vi "ShoulderBegin.vi"(8 "error in (no error)":errorcluster) -> (0 "error out":errorcluster)   [LabVIEW 2023]
doc: "Arm begin\nOpens ArmLift motor\nInputs:\nNone\nOutputs:\nnone"
uses:
  <vilib>/Rock Robotics/WPI/ThirdParty/REV Robotics/REVLib/Typedef/Spark MAX Sensor Type.ctl
  <vilib>/Rock Robotics/WPI/ThirdParty/REV Robotics/REVLib/Typedef/Spark MAX Limit Direction.ctl
  <vilib>/Rock Robotics/WPI/ThirdParty/REV Robotics/REVLib/Typedef/Spark MAX Limit Switch Polarity.ctl
  <vilib>/Rock Robotics/WPI/ThirdParty/REV Robotics/REVLib/Typedef/Spark MAX Idle Mode.ctl
  <vilib>/Rock Robotics/WPI/ThirdParty/REV Robotics/REVLib/Typedef/Spark MAX Motor Type.ctl
  <vilib>/Rock Robotics/WPI/Switch/WPI_SwitchOpenLimit.vi
  <vilib>/Rock Robotics/SystemInterfaces/DIO/FPGA_DIOChannel.ctl
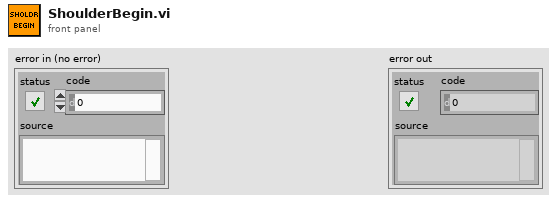
[diagram p1: front panel]
types:
  T1 = typedef "Spark MAX Sensor Type.ctl" = enum16{"No Sensor", "Hall Sensor", "Encoder", "-Not Available-", "Analog", "Alternate Encoder", "Duty Cycle"}
  T2 = typedef "Spark MAX Limit Switch Polarity.ctl" = enum16{"Normally Open", "Normally Closed"}
  T3 = typedef "Spark MAX Limit Direction.ctl" = enum16{"Forward Limit", "Reverse Limit"}
  T4 = typedef "Spark MAX Idle Mode.ctl" = enum16{"Coast", "Brake"}
  T5 = typedef "Spark MAX Motor Type.ctl" = enum16{"Brushed", "Brushless"}
  T6 = typedef "WPI_MotorControlDeviceRef.ctl" = cluster{"DeviceStatus":errorcluster, "Type":T7, "PWM":cluster{"PWM Channel":T8, "DeadBand":T9}, "CAN":cluster{"Device Number":u8, "SetOutput VI Ref":variant, "GetOutput VI Ref":variant, "Enable VI Ref":variant, "Disable VI Ref":variant, "Data":variant}, "Invert":bool, "DIO PWM":cluster{"PWM \"Enable\" Channel":T8, "DIOChannel":T10, "PWM Rate":dbl}}
  T7 = typedef "WPI_MotorControlType.ctl" = enum16{"PWM", "CAN", "DIO PWM"}
  T8 = typedef "FPGA_DIOPWMChannel.ctl" = enum8{"PWM 0", "PWM 1", "PWM 2", "PWM 3", "PWM 4", "PWM 5", "PWM 6", "PWM 7", "PWM 8", "PWM 9", "PWM MXP 0", "PWM MXP 1", "PWM MXP 2", "PWM MXP 3", "PWM MXP 4", "PWM MXP 5", "PWM MXP 6", "PWM MXP 7", "PWM MXP 8", "PWM MXP 9", "Invalid"}
  T9 = typedef "WPI_PWMDeadband.ctl" = cluster{"Name":string, "maxPositivePwm":i32, "minPositivePwm":i32, "centerPwm":i32, "maxNegativePwm":i32, "minNegativePwm":i32, "angularRange":u16}
  T10 = typedef "FPGA_DIOChannel.ctl" = enum8{"DIO 0", "DIO 1", "DIO 2", "DIO 3", "DIO 4", "DIO 5", "DIO 6", "DIO 7", "DIO 8", "DIO 9", "DIO MXP 0", "DIO MXP 1", "DIO MXP 2", "DIO MXP 3", "DIO MXP 4", "DIO MXP 5", "DIO MXP 6", "DIO MXP 7", "DIO MXP 8", "DIO MXP 9", "DIO MXP 10", "DIO MXP 11", "DIO MXP 12", "DIO MXP 13", "DIO MXP 14", "DIO MXP 15", "SPI Port CS1", "SPI Port CS2", "SPI Port CS3", "SPI Port MISO", "SPI Port MOSI", "Invalid"}
  T11 = typedef "WPI_SwitchDevRef.ctl" = cluster{"DevStatus":errorcluster, "DIO Channel":T10, "CntIndex":T12, "Normally Closed":bool}
  T12 = typedef "FPGA_CounterCtrSystemIndex.ctl" = enum8{"Ctr 0", "Ctr 1", "Ctr 2", "Ctr 3", "Ctr 4", "Ctr 5", "Ctr 6", "Ctr 7", "Invalid"}
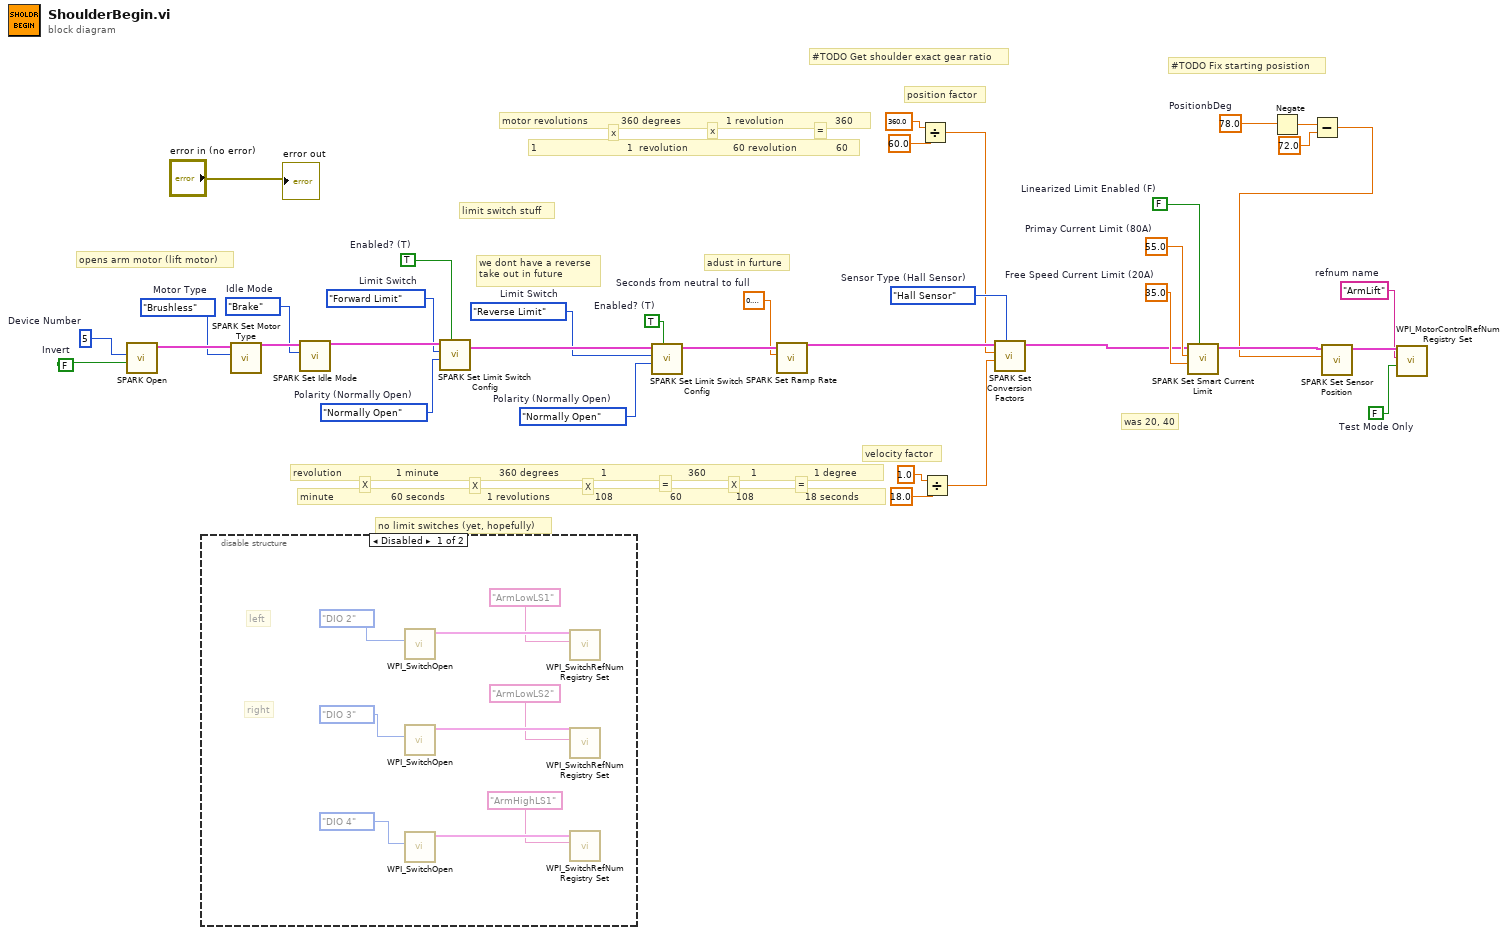
[diagram p0: block diagram]
diagram:
  w8 = FALSE  # Test Mode Only
  w13 = FALSE  # Linearized Limit Enabled (F)
  w15 = Spark_MAX_Sensor_Type."Hall Sensor"  # Sensor Type (Hall Sensor)
  w17 = sgl 0.2  # Seconds from neutral to full
  w19 = Spark_MAX_Limit_Switch_Polarity."Normally Open"  # Polarity (Normally Open)
  w20 = TRUE  # Enabled? (T)
  w21 = Spark_MAX_Limit_Direction."Reverse Limit"  # Limit Switch
  w23 = Spark_MAX_Limit_Switch_Polarity."Normally Open"  # Polarity (Normally Open)
  w24 = TRUE  # Enabled? (T)
  w25 = Spark_MAX_Limit_Direction."Forward Limit"  # Limit Switch
  w4 = 78.0  # PositionbDeg
  w27 = "ArmLift"  # refnum name
  w30 = 35.0  # Free Speed Current Limit (20A)
  w31 = 55.0  # Primay Current Limit (80A)
  w32 = Spark_MAX_Idle_Mode."Brake"  # Idle Mode
  w34 = Spark_MAX_Motor_Type."Brushless"  # Motor Type
  w36 = FALSE  # Invert
  w37 = u8 5  # Device Number
  # "#TODO Get shoulder exact gear ratio"
  # "#TODO Fix starting posistion"
  # "no limit switches (yet, hopefully)"
  # "was 20, 40"
  # "we dont have a reverse\ntake out in future"
  # "adust in furture"
  # "velocity factor"
  # "position factor"
  # "limit switch stuff"
  # "X"
  # "X"
  # "X"
  # "X"
  # "="
  # "="
  # "minute                   60 seconds              1 revolutions               108                   60                  108                 18 seconds"
  # "revolution                  1 minute                    360 degrees              1                           360               1                   1 degree"
  # "1                              1  revolution               60 revolution             60"
  # "="
  # "x"
  # "x"
  # "motor revolutions           360 degrees               1 revolution                 360"
  # "opens arm motor (lift motor)"
  n1 = call <vilib>:"SPARK Open.vi"("Invert"=w36, "Device Number"=w37) -> ("MotorControlDeviceRef"=w35:T6)  [unwired: 8 in, 1 out]
  n2 = disable-structure shown="Disabled" {
    frame Disabled {
      # "right"
      # "left"
      n3 = call-poly <vilib>:"WPI_SwitchOpen.vi"("DIO Channel"=FPGA_DIOChannel."DIO 2") -> ("SwitchDevRef"=w46:T11)  [unwired: 9 in, 1 out]
      n4 = call-poly <vilib>:"WPI_SwitchOpen.vi"("DIO Channel"=FPGA_DIOChannel."DIO 3") -> ("SwitchDevRef"=w40:T11)  [unwired: 9 in, 1 out]
      n5 = call-poly <vilib>:"WPI_SwitchOpen.vi"("DIO Channel"=FPGA_DIOChannel."DIO 4") -> ("SwitchDevRef"=w43:T11)  [unwired: 9 in, 1 out]
      n6 = call <vilib>:"WPI_SwitchRefNum Registry Set.vi"("refnum name"="ArmLowLS1", "SwitchDevRef"=w46) -> ()  [unwired: 8 in, 2 out]
      n7 = call <vilib>:"WPI_SwitchRefNum Registry Set.vi"("refnum name"="ArmLowLS2", "SwitchDevRef"=w40) -> ()  [unwired: 8 in, 2 out]
      n8 = call <vilib>:"WPI_SwitchRefNum Registry Set.vi"("refnum name"="ArmHighLS1", "SwitchDevRef"=w43) -> ()  [unwired: 8 in, 2 out]
    }
    frame Enabled {
    }
  }
  n9 = call <vilib>:"SPARK Set Motor Type.vi"("Motor Type"=w34, "MotorControlDevRef"=w35) -> ("MotorControlDeviceRef"=w33:T6)  [unwired: 8 in, 1 out]
  n10 = call <vilib>:"SPARK Set Idle Mode.vi"("Idle Mode"=w32, "MotorControlDeviceRef in"=w33) -> ("MotorControlDeviceRef out"=w26:T6)  [unwired: 8 in, 1 out]
  n11 = call <vilib>:"SPARK Set Limit Switch Config.vi"("Enabled? (T)"=w24, "Polarity (Normally Open)"=w23, "Limit Switch"=w25, "MotorControlDeviceRef in"=w26) -> ("MotorControlDeviceRef out"=w22:T6)  [unwired: 6 in, 1 out]
  n12 = call <vilib>:"SPARK Set Limit Switch Config.vi"("Enabled? (T)"=w20, "Polarity (Normally Open)"=w19, "Limit Switch"=w21, "MotorControlDeviceRef in"=w22) -> ("MotorControlDeviceRef out"=w18:T6)  [unwired: 6 in, 1 out]
  n13 = call <vilib>:"SPARK Set Ramp Rate.vi"("Seconds from neutral to full (0)"=w17, "MotorControlDeviceRef in"=w18) -> ("MotorControlDeviceRef"=w16:T6)  [unwired: 8 in, 1 out]
  n14 = Divide(x=360.0 ("Velocity Factor (1)"), y=60.0) -> (x/y=w6:dbl)
  n15 = Divide(x=1.0 ("Velocity Factor (1)"), y=18.0) -> (x/y=w5:dbl)
  n16 = call <vilib>:"SPARK Set Conversion Factors.vi"("Sensor Type (Hall Sensor)"=w15, "Velocity Factor (1)"=w5, "Position Factor (1)"=w6, "MotorControlDeviceRef in"=w16) -> ("MotorControlDeviceRef out"=w14:T6)  [unwired: 6 in, 1 out]
  n17 = call <vilib>:"SPARK Set Smart Current Limit.vi"("Linearized Limit Enabled (F)"=w13, "Free Speed Current Limit (20A)"=w30, "Primay Current Limit (80A)"=w31, "MotorControlDeviceRef in"=w14) -> ("MotorControlDeviceRef out"=w29:T6)  [unwired: 6 in, 1 out]
  n18 = Negate(x=w4) -> (-x=w3:dbl)
  n19 = Subtract(x=w3, y=72.0) -> (x-y=w1:dbl)
  n20 = call <vilib>:"SPARK Set Sensor Position.vi"("Position"=w1, "MotorControlDeviceRef"=w29) -> ("MotorControlDeviceRef"=w28:T6)  [unwired: 8 in, 1 out]
  n21 = call <vilib>:"WPI_MotorControlRefNum Registry Set.vi"("Test Mode Only"=w8, "refnum name"=w27, "MotorControlDevRef"=w28) -> ()  [unwired: 7 in, 2 out]
  "error out" <- "error in (no error)"
